vi "Name from Source.vi"(3 "Source":string) -> (1 "Name":string)   [LabVIEW 2020, in "GPack.lvlib" / "GitPackage.lvclass"]
uses:
  GitPackage.lvclass
  <vilib>/regexp/Match Regular Expression.xnode
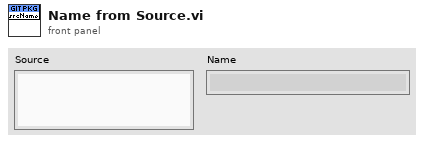
[diagram p1: front panel]
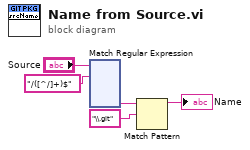
[diagram p0: block diagram]
diagram:
  n1 = xnode "Match Regular Expression"("input string"="Source", "regular expression"="/([^/]+)$") -> ("submatch 1"=w3:string)  [unwired: 4 in, 5 out]
  n2 = Match Pattern(string=w3, regular expression="\\.git") -> (before substring=→"Name":string)  [unwired: 1 in, 3 out]
